vi "CRYGet Global Buffer.vi"(0 "Chn Idx":u32) -> (7 "Global Buffer Out":sgl[](array[numeric]), 10 "isEmpty":bool)   [LabVIEW 2013]
uses:
  CRYMisc vis settings global.vi
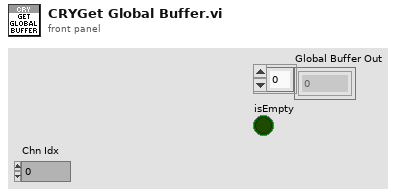
[diagram p1: front panel]
types:
  T1 = cluster{"Gen Idx":i32, "Chn Idx":i32, "Data":sgl[]}[]
  T2 = cluster{"Gen Idx":i32, "Chn Idx":i32, "Data":sgl[]}
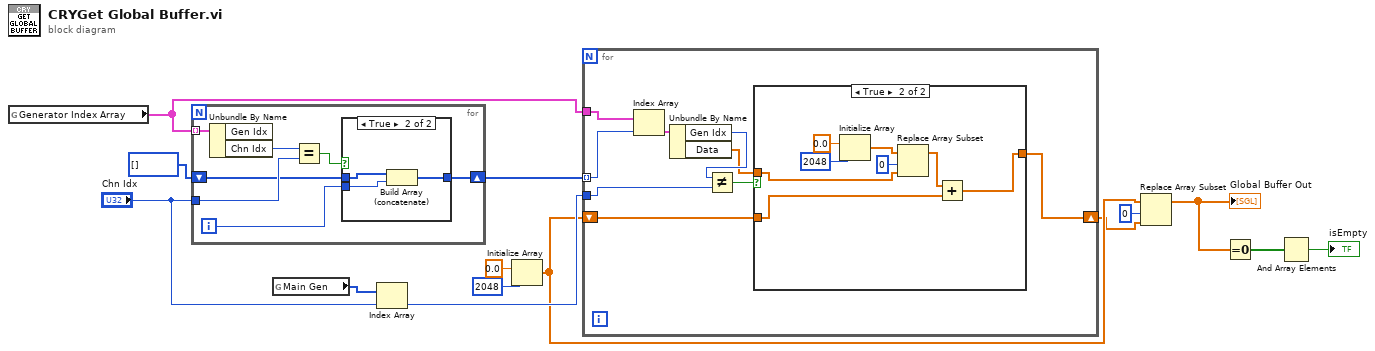
[diagram p0: block diagram]
diagram:
  n1 = global read "CRYMisc vis settings global.vi" "Generator Index Array"() -> (w10:T1)
  n2 = for {
    tunnel: w10 -> [w21] mode=indexing
    tunnel: "Chn Idx" -> [w20]
    shift-right: [w16] -> w11
    shift-left: i32[] [] -> [w15]
    i -> [w17]
    n3 = Unbundle By Name(w21) -> ("Chn Idx"=w19:i32)  [unwired: 1 out]
    n4 = Equal?(x=w19, y=w20) -> (x = y?=w18:bool)
    n5 = case shown="True" w18 {
      tunnel: w17 -> [_ w25]
      tunnel: [w22 w24] -> w16
      tunnel: w15 -> [w22 w23]
      frame False {
      }
      frame True {
        n6 = Build Array (concatenate)(w23, w25) -> (w24:i32[])
      }
    }
  }
  n7 = global read "CRYMisc vis settings global.vi" "Main Gen"() -> (w13:i32[])
  n8 = Index Array(array=w13, index="Chn Idx") -> (element=w9:i32)
  n9 = Initialize Array(sgl 0.0 ("element"), 2048 ("dimension size")) -> (w5:sgl[])
  n10 = for {
    tunnel: w11 -> [w33] mode=indexing
    tunnel: w10 -> [w34]
    tunnel: w9 -> [w29]
    shift-right: [w27] -> w4
    shift-left: w5 -> [w26]
    n11 = Index Array(array=w34, index=w33) -> (element=w32:T2)
    n12 = Unbundle By Name(w32) -> ("Gen Idx"=w30:i32, "Data"=w28:sgl[])
    n13 = Not Equal?(x=w30, y=w29) -> (x != y?=w31:bool)
    n14 = case shown="True" w31 {
      tunnel: w28 -> [_ w39]
      tunnel: [w35 w36] -> w27
      tunnel: w26 -> [w35 w37]
      frame False {
      }
      frame True {
        n15 = Initialize Array(sgl 0.0 ("element"), 2048 ("dimension size")) -> (w40:sgl[])
        n16 = Replace Array Subset(array=w40, new element=w39, index=0) -> (w38:sgl[])
        n17 = Add(x=w38, y=w37) -> (x+y=w36:sgl[])
      }
    }
  }
  n18 = Replace Array Subset(array=w5, new element=w4, index=0) -> (w2:sgl[])
  "Global Buffer Out" <- w2
  n19 = Equal To 0?(x=w2) -> (x = 0?=w3:bool[])
  n20 = And Array Elements(Boolean array=w3) -> (logical AND=→"isEmpty":bool)
